vi "LV86_Median.vi"(3 "Image in":T2 {"Dialogs" format="%.0b"}) -> (1 "Image out":T2 {"Dialogs" format="%.0b"})   [LabVIEW 2024]
doc: "This VI applies a median filter to the image"
uses:
  <userlib>/ImageProcessing/QTLIB_2595_LV86/QT_Image.ctl
panel:
  in  "Size & Order #":T1={"X Size"=3, "Y Size"=3, "Order #"=4}
  # "This VI applies a median filter to the image"
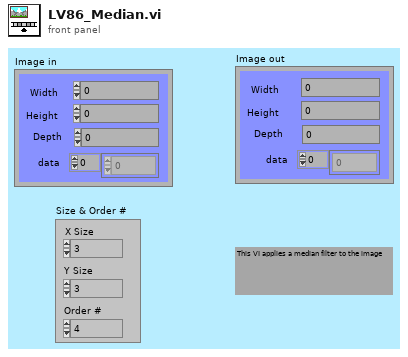
[diagram p1: front panel]
types:
  T1 = cluster{"X Size":i32, "Y Size":i32, "Order #":i32}
  T2 = typedef "QT_Image.ctl" = cluster{"Width":i32, "Height":i32, "Depth":i32, "data":u8[], "Compressed data":u8[], "Color table":u32[], "Duration":i32, "Options":i32, "Timestamp":i32, "ID":i32, "Reserved":i32, "Dialogs":u32}
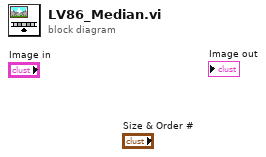
[diagram p0: block diagram]
diagram:
